vi "AWGSendPulseArray.vi"(8 "error in (no error)":errorcluster, 10 "Step Number":i32, 11 "AWG pulses array":variant[](array[variant])) -> (0 "error out":errorcluster)   [LabVIEW 2019]
panel:
  in  "Sample rate":dbl=500000000.0 format="%^#_6g"
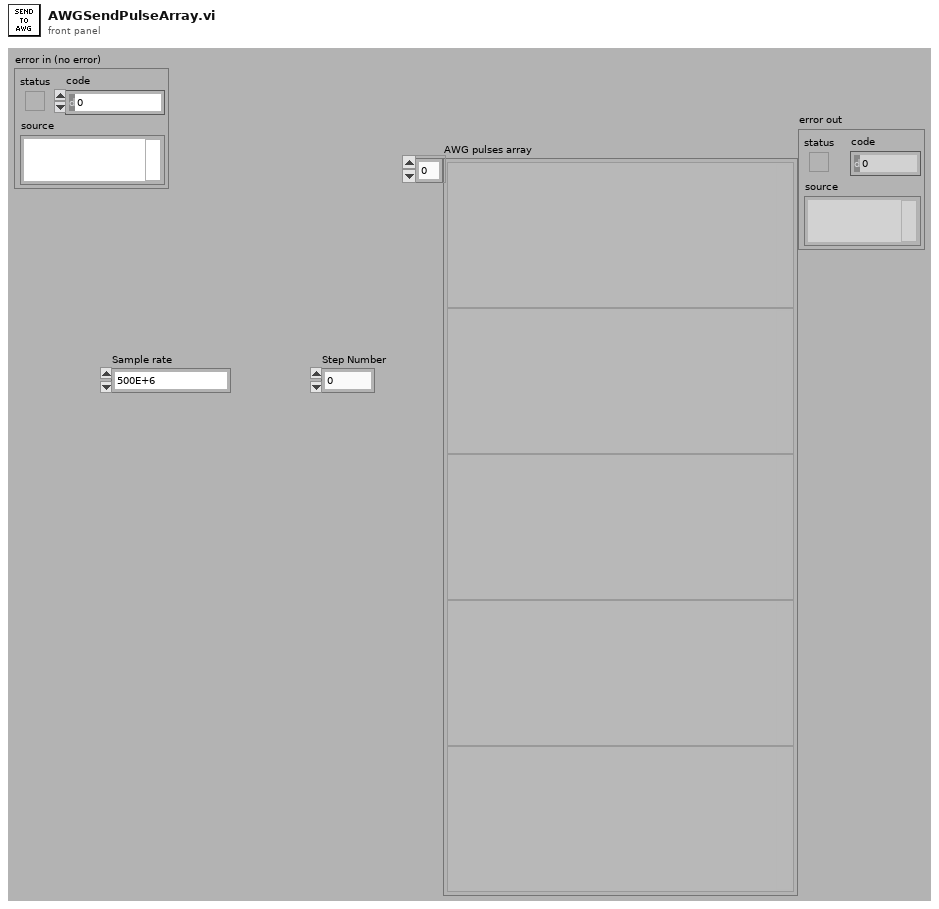
[diagram p1: front panel]
types:
  T1 = cluster{"Sample rate":dbl, "Step Number":i32, "Array":variant[], "mVpp":dbl}
  T2 = cluster{"Sample rate":dbl, "Step Number":i32, "AWG pulses array":variant[], dbl}
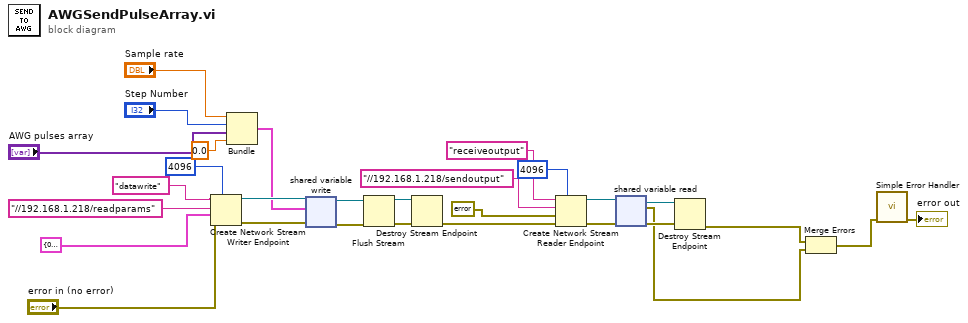
[diagram p0: block diagram]
diagram:
  n1 = Create Network Stream Writer Endpoint(7:4096 ("writer buffer size"), 8:"error in (no error)", 9:T1 {"Sample rate"=0.0, "Step Number"=0, "Array"=[], "mVpp"=0.0} ("output cluster"), 10:"//192.168.1.218/readparams" ("reader url"), 11:"datawrite" ("writer name")) -> (0:w19:errorcluster, 3:w20:refnum<k21>)  [unwired: 2 in]
  n2 = Bundle("Sample rate"="Sample rate", "Step Number"="Step Number", "AWG pulses array"="AWG pulses array", 0.0) -> (w12:T2)  [unwired: 1 in]
  n3 = shared-variable-write(w20, w19, w12) -> (w18:refnum<k21>, w17:errorcluster)  [unwired: 1 in, 1 out]
  n4 = Flush Stream(8:w17, 11:w18) -> (0:w29:errorcluster, 3:w28:refnum<k21>)  [unwired: 2 in, 1 out]
  n5 = Destroy Stream Endpoint(8:w29, 11:w28) -> (0:w9:errorcluster)
  n6 = Create Network Stream Reader Endpoint(7:4096 ("reader buffer size"), 8:w9, 9:errorcluster {"status"=FALSE, "code"=0, "source"=""} ("error out"), 10:"//192.168.1.218/sendoutput" ("writer url"), 11:"receiveoutput" ("reader name")) -> (0:w25:errorcluster, 3:w26:refnum<k21>)  [unwired: 2 in]
  n7 = shared-variable-read(w26, w25) -> (w24:refnum<k21>, w23:errorcluster, w3:errorcluster)  [unwired: 1 in, 1 out]
  n8 = Destroy Stream Endpoint(8:w23, 11:w24) -> (0:w8:errorcluster)
  n9 = Merge Errors(w8, w3) -> (w7:errorcluster)
  n10 = call <vilib>:"Simple Error Handler.vi"("error in (no error)"=w7) -> ("error out"=→"error out":errorcluster)  [unwired: 4 in, 4 out]
